vi "CRYAPI Pic ChangeActiveWinTitle.vi"(11 "tFrame":T2) -> ()   [LabVIEW 2013]
uses:
  <vilib>/Utility/miscctls.llb/LVRectTypeDef.ctl
  CRYMain Sub Window Global.vi
  CRYStepSetup/CRYStepSetup Global.vi
panel:
  in  "bWait":bool=TRUE
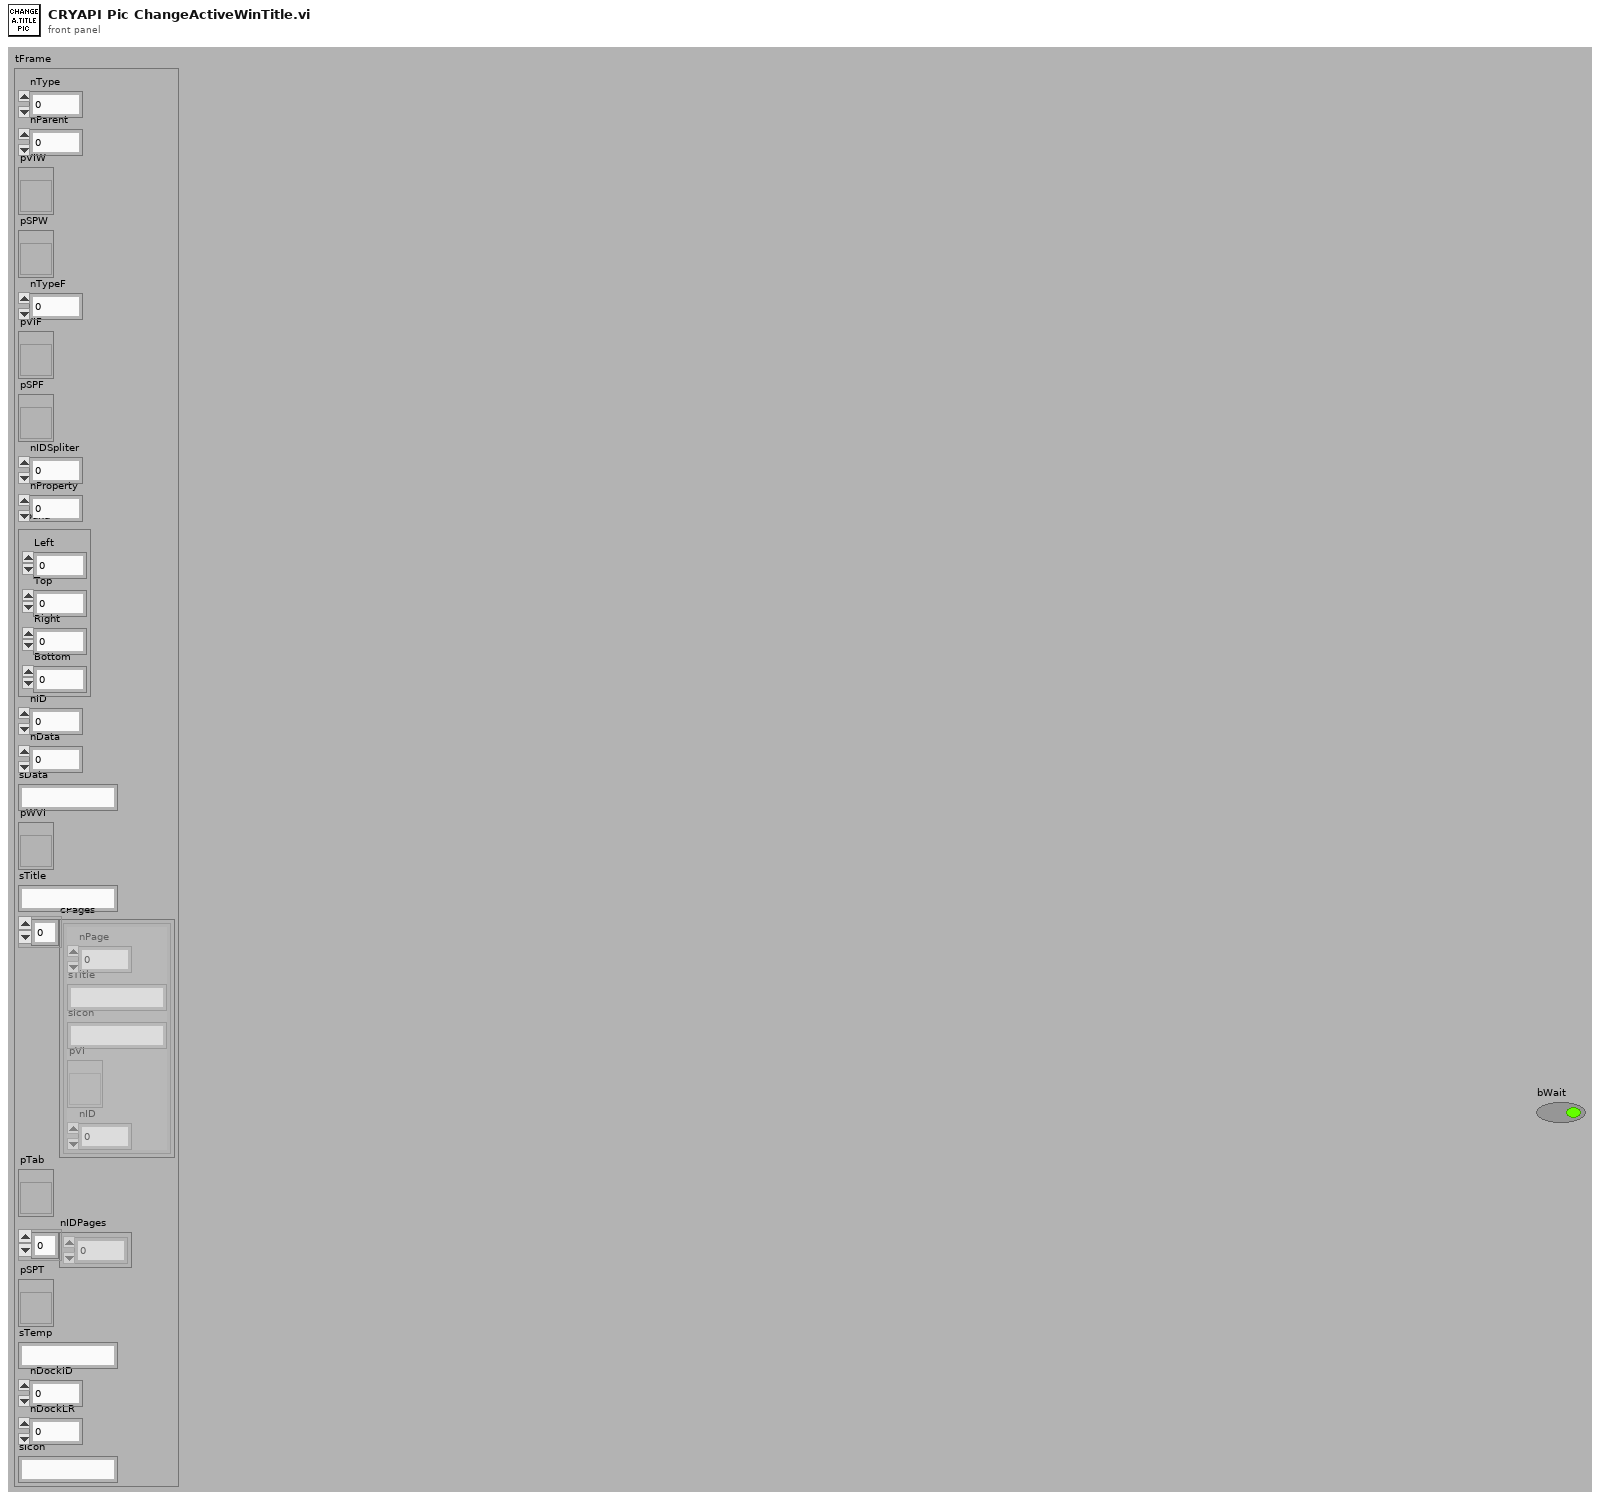
[diagram p1: front panel]
types:
  T1 = typedef "LVRectTypeDef.ctl" = cluster{"Left":i16, "Top":i16, "Right":i16, "Bottom":i16}
  T2 = cluster{"nType":i32, "nParent":i32, "pVIW":refnum<vi>, "pSPW":refnum<vi>, "nTypeF":i32, "pVIF":refnum<vi>, "pSPF":refnum<vi>, "nIDSpliter":i32, "nProperty":i32, "Bound":T1, "nID":i32, "nData":i32, "sData":string, "pWVI":refnum<vi>, "sTitle":string, "cPages":cluster{"nPage":i32, "sTitle":string, "sIcon":string, "pVI":refnum<vi>, "nID":i32}[], "pTab":refnum<vi>, "nIDPages":i32[], "pSPT":refnum<vi>, "sTemp":string, "nDockID":i32, "nDockLR":i32, "sIcon":string}
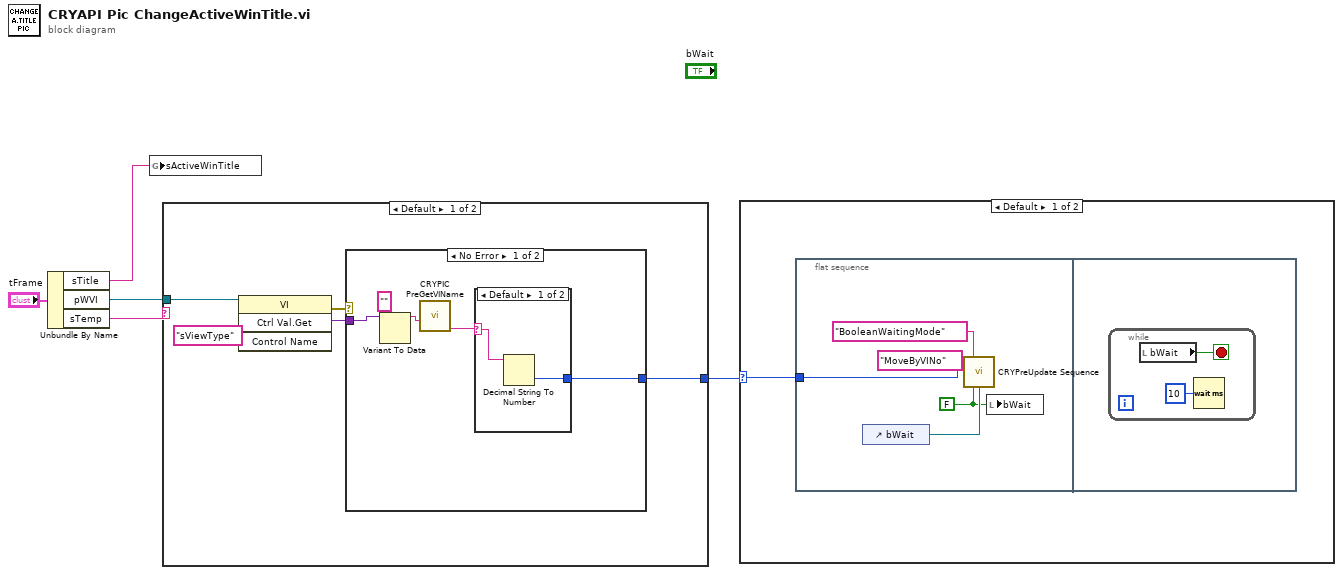
[diagram p0: block diagram]
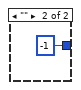
[diagram p3: hidden frame]
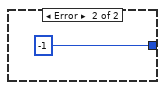
[diagram p4: hidden frame]
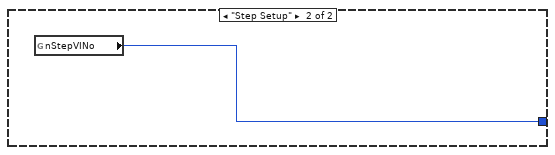
[diagram p5: hidden frame]
diagram:
  n1 = Unbundle By Name("tFrame") -> ("sTitle"=w2:string, "pWVI"=w3:refnum<vi>, "sTemp"=w4:string)
  n2 = global write "CRYMain Sub Window Global.vi" "sActiveWinTitle"(w2) -> ()
  n3 = case shown="Default" w4 {
    tunnel: w3 -> [w10 _]
    tunnel: [w6 w20] -> w1
    frame Default {
      n4 = invoke class="VI" method="Ctrl Val.Get"(reference=w10, "Control Name"="sViewType") -> (error out=w8:errorcluster, "Get Control Value Variant"=w7:variant)  [unwired: 2 in, 2 out]
      n5 = case shown="No Error" w8 {
        tunnel: w7 -> [w15 _]
        tunnel: [w12 -1] -> w6
        frame No Error {
          n6 = Variant To Data(type="", Variant=w15) -> (data=w13:string)  [unwired: 1 in, 1 out]
          n7 = call "CRYPIC PreGetVIName.vi"("sVIName"=w13) -> ("sData_Out"=w11:string)  [unwired: 9 in, 1 out]
          n8 = case shown="Default" w11 {
            selector: w11 -> [w16 _]
            tunnel: [w17 -1] -> w12
            frame Default {
              n9 = Decimal String To Number(string=w16) -> (number=w17:i32)  [unwired: 2 in, 1 out]
            }
            frame "" {
            }
          }
        }
        frame Error {
        }
      }
    }
    frame "Step Setup" {
      n10 = global read "CRYStepSetup Global.vi" "nStepVINo"() -> (w20:i32)
    }
  }
  n11 = case shown="Default" w1 {
    selector: w1 -> [w21 _]
    frame Default {
      n12 = flat-sequence {
        tunnel: w21 -> [w22]
        frame #0 {
          w25 = FALSE ("AllChangeFlg")
          n13 = control-ref of="bWait"() -> (w26:refnum<vi>)
          n14 = call "CRYPreUpdate Sequence.vi"("EventName"="MoveByVINo", "Mode"="BooleanWaitingMode", "Proper VI No"=w22, "AllChangeFlg"=w25, "Ref Variant"=w26) -> ()  [unwired: 11 in]
          n15 = local write "bWait"(w25) -> ()
        }
        frame #1 {
          n16 = while {
            stop <- w28 stop-if-true
            n17 = local read "bWait"() -> (w28:bool)
            n18 = Wait (ms)(milliseconds to wait=u32 10) -> ()  [unwired: 1 out]
          }
        }
      }
    }
    frame -1 {
    }
  }
